vi "Cell V Set.vi"(7 "Box ID":u8=1, 8 "error in (no error)":errorcluster, 9 "Voltage":dbl, 10 "Channel":u16, 11 "CAN in":refnum<class "XNET_BS120x.lvclass">) -> (0 "error out":errorcluster, 3 "CAN out":refnum<class "XNET_BS120x.lvclass">)   [LabVIEW 2021, in "BS120x Driver.lvlib" / "XNET_BS120x.lvclass"]
uses:
  XNET_BS120x.lvclass
  BS120x.lvclass
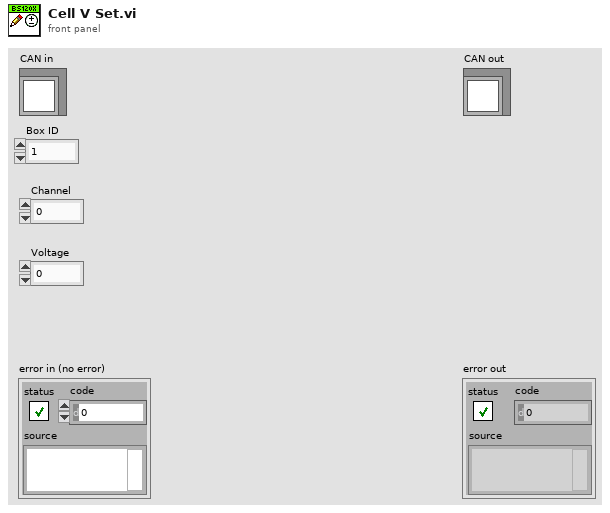
[diagram p1: front panel]
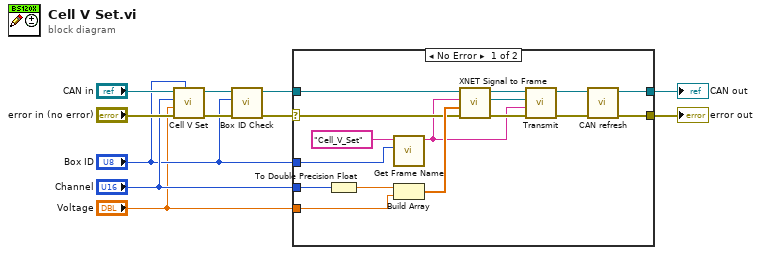
[diagram p0: block diagram]
diagram:
  n1 = call-parent "Cell V Set.vi"("Box ID"="Box ID", "error in (no error)"="error in (no error)", "Voltage"="Voltage", "Channel"="Channel", "BS120x in"="CAN in") -> ("error out"=w6:errorcluster, "BS120x out"=w5:refnum<class "XNET_BS120x.lvclass">)  [unwired: 5 in]
  n2 = call "Box ID Check.vi"("error in (no error)"=w6, "Box ID"="Box ID", "CAN in"=w5) -> ("error out"=w8:errorcluster, "CAN out"=w9:refnum<class "XNET_BS120x.lvclass">)  [unwired: 7 in]
  n3 = case shown="No Error" w8 {
    selector: w8 -> [w14 w28]
    tunnel: "Channel" -> [w26 _]
    tunnel: w9 -> [w25 w29]
    tunnel: [w19 w28] -> w11
    tunnel: [w17 w29] -> w10
    tunnel: "Box ID" -> [w15 _]
    tunnel: "Voltage" -> [w13 _]
    frame No Error {
      n4 = To Double Precision Float(number=w26) -> (double precision float=w27:dbl)
      n5 = call "Get Frame Name.vi"("Box ID"=w15, "Frame Name"="Cell_V_Set" ("Frame")) -> ("Frame Name out"=w12:string)  [unwired: 9 in]
      n6 = Build Array(w27, w13) -> (w24:dbl[])
      n7 = call "XNET Signal to Frame.vi"("error in (no error)"=w14, "Data Array"=w24, "Frame"=w12, "CAN in"=w25) -> ("error out"=w21:errorcluster, "Data"=w22:refnum<class "XNET Data.lvclass">, "CAN out"=w23:refnum<class "XNET_BS120x.lvclass">)  [unwired: 5 in]
      n8 = call "Transmit.vi"("error in (no error)"=w21, "Frame"=w12, "Data in"=w22, "CAN in"=w23) -> ("error out"=w20:errorcluster, "CAN out"=w18:refnum<class "XNET_BS120x.lvclass">)  [unwired: 6 in]
      n9 = call "CAN refresh.vi"("error in (no error)"=w20, "CAN in"=w18) -> ("error out"=w19:errorcluster, "CAN out"=w17:refnum<class "XNET_BS120x.lvclass">)  [unwired: 8 in]
    }
    frame Error {
    }
  }
  "error out" <- w11
  "CAN out" <- w10
